vi "read_decrypted_Password.vi"(9 "Password":string, 10 "error in":errorcluster, 11 "Username":string) -> (3 "Username 2":string, 4 "error Out":errorcluster, 5 "Decrypted":string)   [LabVIEW 2013]
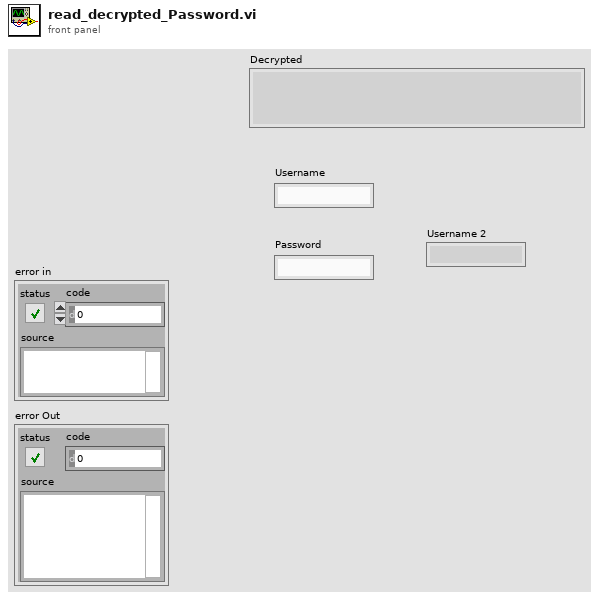
[diagram p1: front panel]
types:
  T1 = enum16{"open", "replace", "create", "open or create", "replace or create", "replace or create with confirmation"}
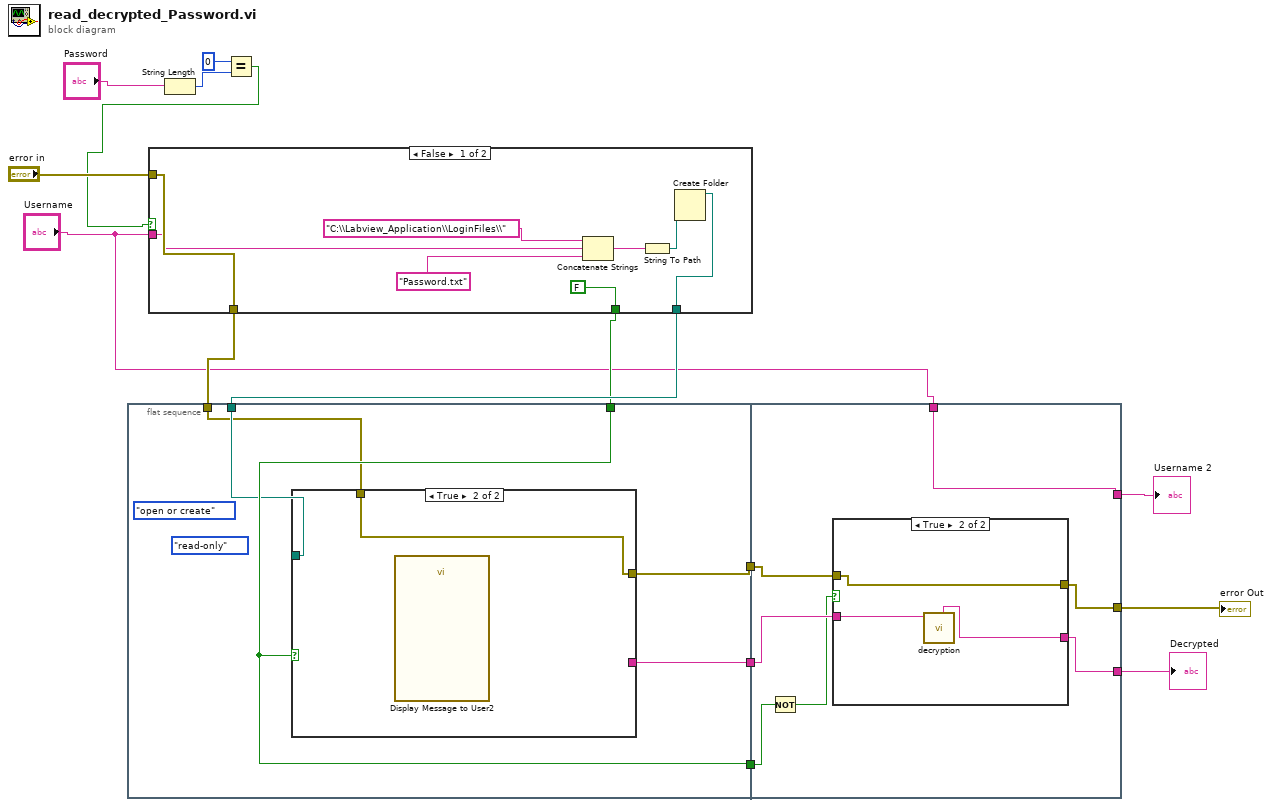
[diagram p0: block diagram]
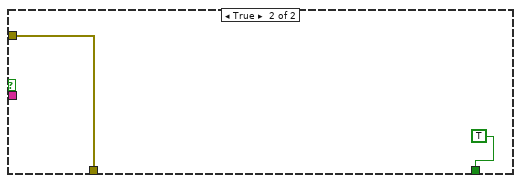
[diagram p2: hidden frame]
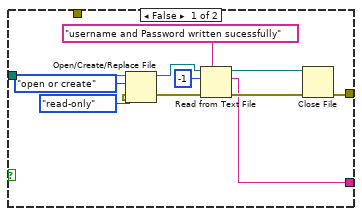
[diagram p3: hidden frame]
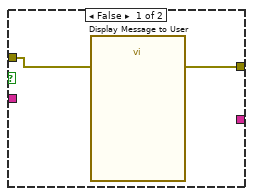
[diagram p4: hidden frame]
diagram:
  n1 = flat-sequence {
    tunnel: w15 -> [w17]
    tunnel: [w20] -> w14
    tunnel: [w19] -> w13
    tunnel: [w18] -> w10
    tunnel: w6 -> [w16]
    tunnel: w4 -> [w18]
    tunnel: w14 -> [w37]
    tunnel: w13 -> [w38]
    tunnel: [w36] -> w12
    tunnel: [w35] -> w11
    tunnel: w10 -> [w34]
    tunnel: "Username" -> [w32]
    tunnel: [w32] -> w1
    frame #0 {
      (unwired) enum16{"read/write", "read-only", "write-only"}."read-only" ("access (0:read/write)")
      (unwired) T1."open or create" ("operation (0:open)")
      n2 = case shown="True" w18 {
        tunnel: [w29 w31] -> w20
        tunnel: [w28 _] -> w19
        tunnel: w17 -> [w24 _]
        tunnel: w16 -> [_ w31]
        frame False {
          n3 = Open/Create/Replace File(file path (use dialog)=w24, operation (0:open)=T1."open or create", access (0:read/write)=enum16{"read/write", "read-only", "write-only"}."read-only") -> (refnum out=w26:refnum<file>, error out=w25:errorcluster)  [unwired: 3 in, 1 out]
          n4 = Read from Text File(prompt (Open existing file)="username and Password written sucessfully" ("prompt (Choose or enter file path)"), file (use dialog)=w26, count=-1, error in=w25) -> (refnum out=w21:refnum<file>, text=w28:string, error out=w29:errorcluster)  [unwired: 1 out]
          n5 = Close File(refnum=w21) -> ()  [unwired: 1 in, 2 out]
        }
        frame True {
          n6 = call "Display Message to User2"() -> ()  [unwired: 10 in, 2 out]
        }
      }
    }
    frame #1 {
      n7 = Not(x=w34) -> (.not. x?=w33:bool)
      n8 = case shown="True" w33 {
        tunnel: w38 -> [_ w42]
        tunnel: w37 -> [w39 w40]
        tunnel: [w39 w40] -> w36
        tunnel: [_ w41] -> w35
        frame False {
          n9 = call "Display Message to User"() -> ()  [unwired: 10 in, 2 out]
        }
        frame True {
          n10 = call "decryption.vi"("String to Decrypt"=w42) -> ("Decrypted"=w41:string)  [unwired: 10 in]
        }
      }
    }
  }
  n11 = String Length(string="Password") -> (length=w8:i32)
  n12 = Equal?(x=0, y=w8) -> (x = y?=w3:bool)
  n13 = case shown="False" w3 {
    tunnel: [w43 _] -> w15
    tunnel: [w46 w52] -> w6
    tunnel: "error in" -> [w46 w52]
    tunnel: [FALSE TRUE] -> w4
    tunnel: "Username" -> [w45 _]
    frame False {
      n14 = Concatenate Strings("C:\\Labview_Application\\LoginFiles\\", w45, "Password.txt") -> (w48:string)
      n15 = String To Path(string=w48) -> (path=w44:path)
      n16 = Create Folder(path (use dialog)=w44) -> (created path=w43:path)  [unwired: 2 in, 2 out]
    }
    frame True {
    }
  }
  "error Out" <- w12
  "Decrypted" <- w11
  "Username 2" <- w1
